vi "Update Control.vi"(8 "error in":errorcluster, 11 "BigMAQ in":refnum<class "BigMAQ.lvclass">) -> (0 "error out":errorcluster, 3 "BigMAQ out":refnum<class "BigMAQ.lvclass">)   [LabVIEW 2019, in "BigMAQ.lvclass"]
uses:
  BigMAQ.lvclass
  BigMAQ.lvclass/BigMAQ.ctl
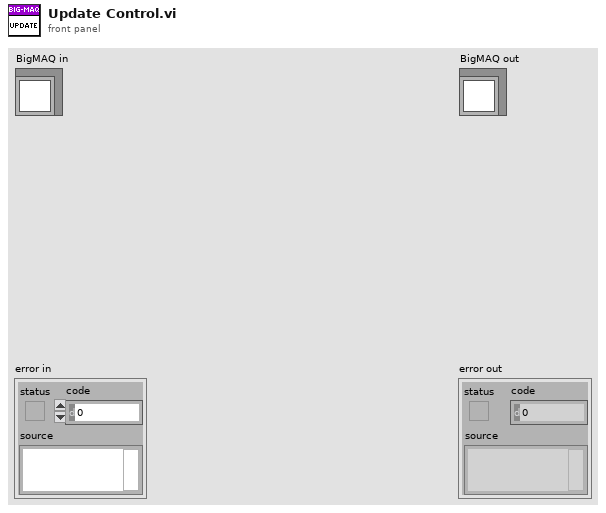
[diagram p1: front panel]
types:
  T1 = typedef "IMAQ Image.ctl" = refnum<image>
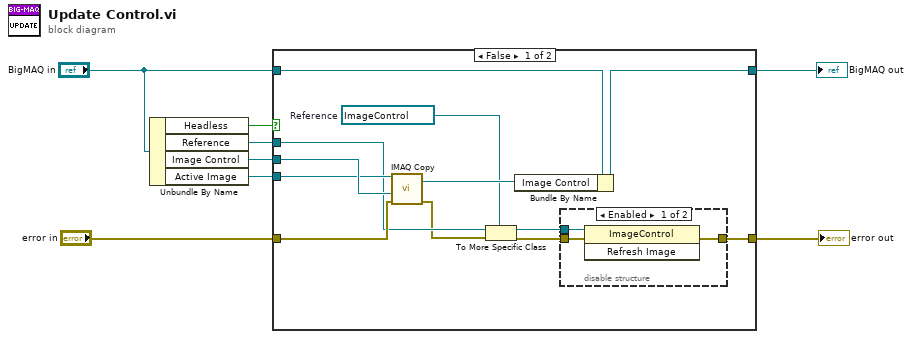
[diagram p0: block diagram]
diagram:
  n1 = Unbundle By Name("BigMAQ in") -> ("Headless"=w1:bool, "Reference"=w8:refnum<vi>, "Image Control"=w6:T1, "Active Image"=w5:T1)
  n2 = case shown="False" w1 {
    tunnel: w8 -> [w11 _]
    tunnel: [w20 w25] -> w7
    tunnel: w6 -> [w19 _]
    tunnel: w5 -> [w18 _]
    tunnel: "error in" -> [w17 w25]
    tunnel: "BigMAQ in" -> [w16 w26]
    tunnel: [w15 w26] -> w2
    frame False {
      w12 = refnum<vi> refnum  # Reference
      n3 = call "IMAQ Copy"("error in (no error)"=w17, "Image Dst"=w19, "Image Src"=w18) -> ("error out"=w10:errorcluster, "Image Dst Out"=w14:T1)  [unwired: 3 in]
      n4 = To More Specific Class(target class=w12, reference=w11, error in=w10) -> (specific class reference=w13:refnum<vi>, error out=w9:errorcluster)
      n5 = Bundle By Name(cluster=w16, "Image Control"=w14) -> (w15:refnum<class "BigMAQ.lvclass">)
      n6 = disable-structure shown="Enabled" {
        disable-tunnel: [w23 w24] -> w20
        disable-tunnel: w13 -> [w22 _]
        disable-tunnel: w9 -> [w21 w24]
        frame Enabled {
          n7 = invoke class="ImageControl" method="Refresh Image"(reference=w22, error in=w21) -> (error out=w23:errorcluster)  [unwired: 1 in, 2 out]
        }
        frame Disabled {
        }
      }
    }
    frame True {
    }
  }
  "error out" <- w7
  "BigMAQ out" <- w2
